vi "Get Shared Library Path.vi"(8 "error in (no error)":errorcluster) -> (0 "error out":errorcluster, 3 "shared library path":path)   [LabVIEW 2020, in "CodeSignAPI.lvlib"]
uses:
  <vilib>/AppBuilder/CodeSignAPI/CodeSignAPI.lvlib
  <vilib>/registry/registry.llb/Registry RtKey.ctl
  <resource>/Framework/Providers/Common/provcom_StringGlobals.vi
  <vilib>/registry/registry.llb/Registry SAM.ctl
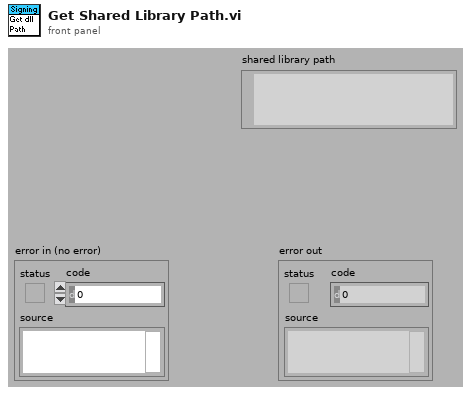
[diagram p1: front panel]
types:
  T1 = typedef "Registry SAM.ctl" = enum32{"KEY_QUERY_VALUE", "KEY_SET_VALUE", "KEY_CREATE_SUB_KEY", "KEY_ENUMERATE_SUB_KEYS", "KEY_NOTIFY", "KEY_CREATE_LINK", "KEY_READ", "KEY_WRITE", "KEY_ALL_ACCESS", "KEY_READ | KEY_WRITE"}
  T2 = typedef "Registry RtKey.ctl" = enum32{"HKEY_CLASSES_ROOT", "HKEY_CURRENT_USER", "HKEY_LOCAL_MACHINE", "HKEY_USERS", "HKEY_PERFORMANCE_DATA", "HKEY_CURRENT_CONFIG", "HKEY_DYN_DATA"}
  T3 = typedef "Registry refnum.ctl" = refnum<k1>
  T4 = cluster{"numValues":i32, "maxValueNameLen":i32, "maxValueDataLen":i32}
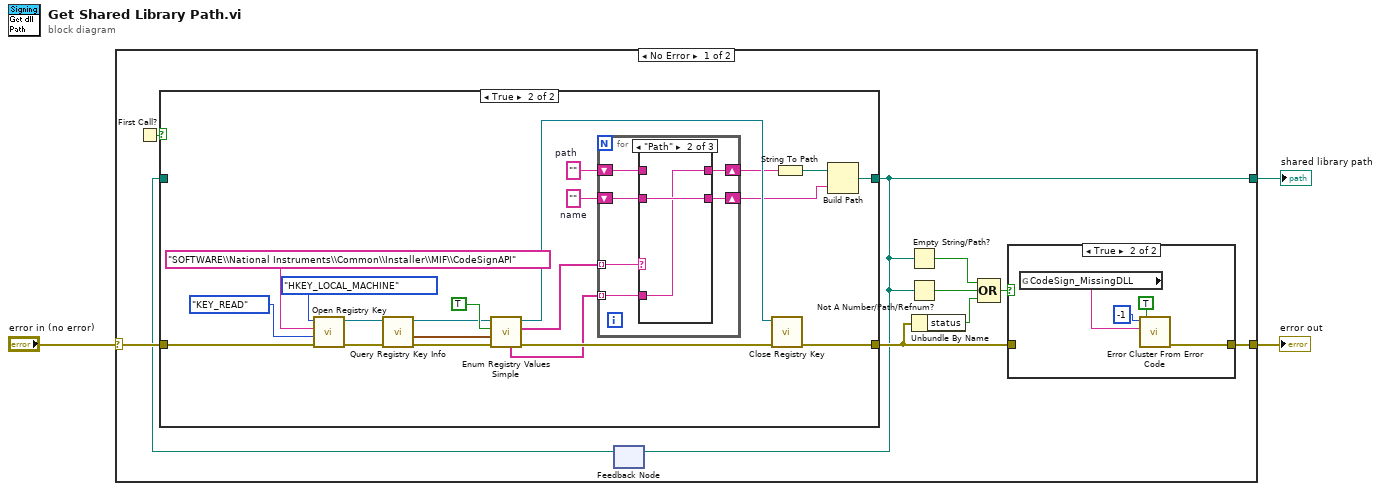
[diagram p0: block diagram]
diagram:
  n1 = case shown="No Error" "error in (no error)" {
    selector: "error in (no error)" -> [w13 w54]
    tunnel: [w10 w54] -> w2
    tunnel: [w4 _] -> w1
    frame No Error {
      n2 = First Call?() -> (First Call?: T/F=w12:bool)
      n3 = feedback #1() -> (w11:path)  [unwired: 1 out]
      n4 = case shown="True" w12 {
        tunnel: w13 -> [w20 w38]
        tunnel: [w20 w37] -> w7
        tunnel: [w19 w30] -> w4
        tunnel: w11 -> [w19 _]
        frame False {
        }
        frame True {
          w31 = ""  # name
          w35 = ""  # path
          n5 = call <vilib>:"Open Registry Key.vi"("error in (no error)"=w38, "security access mask (KEY_READ | KEY_WRITE)"=Registry_SAM."KEY_READ", "subkey"="SOFTWARE\\National Instruments\\Common\\Installer\\MIF\\CodeSignAPI", "root key (HKEY_LOCAL_MACHINE)"=Registry_RtKey."HKEY_LOCAL_MACHINE") -> ("error out"=w24:errorcluster, "refnum out"=w26:T3)  [unwired: 6 out]
          n6 = call <vilib>:"Query Registry Key Info.vi"("error in (no error)"=w24, "refnum"=w26) -> ("error out"=w23:errorcluster, "value info"=w22:T4, "refnum out"=w25:T3)  [unwired: 7 out]
          n7 = call <vilib>:"Enum Registry Values Simple.vi"("error in (no error)"=w23, "value info"=w22, "retrieve data? (F)"=TRUE, "refnum"=w25) -> ("error out"=w33:errorcluster, "values"=w36:string[], "refnum out"=w34:T3, "String/Binary data"=w32:string[])  [unwired: 4 out]
          n8 = for {
            tunnel: w36 -> [w47] mode=indexing
            shift-right: [w43] -> w29
            shift-left: w35 -> [w42]
            shift-right: [w45] -> w27
            shift-left: w31 -> [w44]
            tunnel: w32 -> [w46] mode=indexing
            n9 = case shown="\"Path\"" w47 {
              tunnel: w46 -> [w49 w50 _]
              tunnel: [w49 w51 w52] -> w45
              tunnel: w44 -> [_ w51 w52]
              tunnel: [w48 w50 w53] -> w43
              tunnel: w42 -> [w48 _ w53]
              frame "DllName" {
              }
              frame "Path" {
              }
              frame Default {
              }
            }
          }
          n10 = call <vilib>:"Close Registry Key.vi"("error in (no error)"=w33, "refnum"=w34) -> ("error out"=w37:errorcluster)  [unwired: 5 out]
          n11 = String To Path(string=w29) -> (path=w28:path)
          n12 = Build Path(base path=w28, name or relative path=w27) -> (appended path=w30:path)
        }
      }
      n13 = feedback-in #1(w4) -> ()
      n14 = Empty String/Path?(string/path=w4) -> (empty?=w5:bool)
      n15 = Not A Number/Path/Refnum?(number/path/refnum=w4) -> (NaN/Path/Refnum?=w6:bool)
      n16 = Unbundle By Name(w7) -> ("status"=w8:bool)
      n17 = Compound Arithmetic op=OR(w5, w6, w8) -> (w9:bool)
      n18 = case shown="True" w9 {
        tunnel: [w14 w18] -> w10
        tunnel: w7 -> [w14 _]
        frame False {
        }
        frame True {
          n19 = global read "provcom_StringGlobals.vi" "CodeSign_MissingDLL"() -> (w16:string)
          n20 = call <vilib>:"Error Cluster From Error Code.vi"("show call chain? (False)"=TRUE, "error message (\"\")"=w16, "error code (0)"=-1) -> ("error out"=w18:errorcluster)  [unwired: 1 in, 5 out]
        }
      }
    }
    frame Error {
    }
  }
  "shared library path" <- w1
  "error out" <- w2
